vi "Interpolate_ArrayTable.vi"(9 "Desired_Distance":dbl, 11 "array":dbl[][](array[numeric])) -> (3 "RPM":dbl)   [LabVIEW 2020]
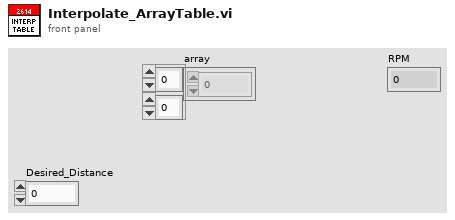
[diagram p1: front panel]
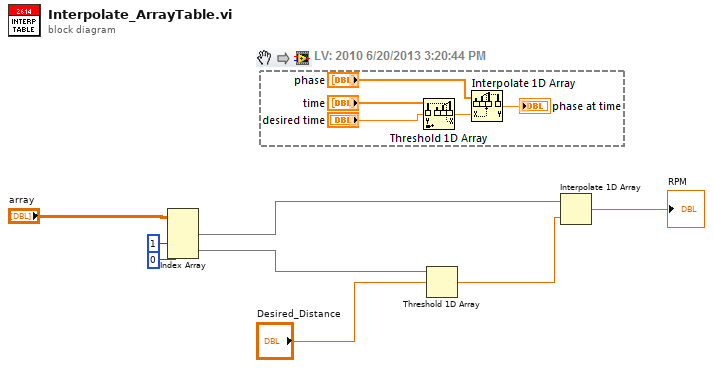
[diagram p0: block diagram]
diagram:
  n1 = Index Array(array="array", index (col) #1=1 ("disabled index (col)"), index (col) #2=0 ("index (col)")) -> (element #1=w4:dbl[], element #2=w3:dbl[])  [unwired: 2 in]
  n2 = Threshold 1D Array(2:"Desired_Distance", 3:w3) -> (0:w6:dbl)  [unwired: 1 in]
  n3 = Interpolate 1D Array(1:w6, 2:w4) -> (0:→"RPM":dbl)
